vi "openVISA_current.vi"(6 "Boolean in":bool, 8 "error in (no error)":errorcluster, 11 "VISA Refnum in":refnum<visa-resource-name>) -> (0 "error out":errorcluster, 3 "VISA Refnum out":refnum<visa-resource-name>, 4 "Boolean out":bool)   [LabVIEW 2026]
uses:
  <vilib>/Instr/_visa.llb/VISA Configure Serial Port (Instr).vi
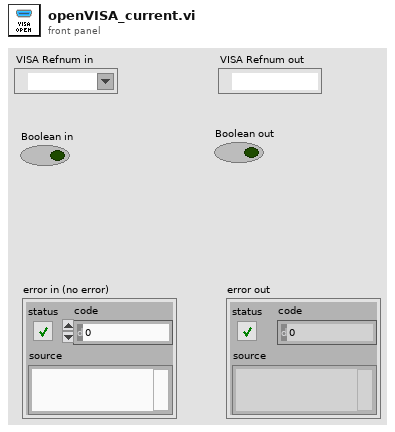
[diagram p1: front panel]
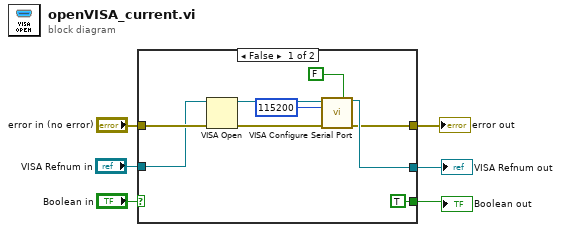
[diagram p0: block diagram]
diagram:
  n1 = case shown="False" "Boolean in" {
    selector: "Boolean in" -> [_ w18]
    tunnel: [TRUE w18] -> w3
    tunnel: "error in (no error)" -> [w10 w17]
    tunnel: [w12 w16] -> w5
    tunnel: [w11 w17] -> w6
    tunnel: "VISA Refnum in" -> [w8 w16]
    frame False {
      n2 = VISA Open(error in (no error)=w10, VISA resource name=w8) -> (VISA resource name=w14:refnum<visa-resource-name>, error out=w15:errorcluster)  [unwired: 3 in]
      n3 = call-poly "VISA Configure Serial Port"("VISA resource name"=w14, "Enable Termination\nChar (T)"=FALSE ("Enable Termination\nChar (T)"), "baud rate (9600)"=u32 115200, "error in (no error)"=w15) -> ("VISA resource name out"=w12:refnum<visa-resource-name>, "error out"=w11:errorcluster)  [unwired: 10 in]
    }
    frame True {
    }
  }
  "error out" <- w6
  "VISA Refnum out" <- w5
  "Boolean out" <- w3
